vi "ORS_Insight_Reduce_B-scan_Data.vi"(4 "length":i32, 6 "offset":i32, 7 "Data Valid Vector":u32[](array[numeric]), 8 "spl per line":i32, 9 "DVV shift":i32, 10 "line Num":i32, 11 "Input":i16[](array[numeric])) -> (3 "Output":i16[](array[numeric]))   [LabVIEW 2024]
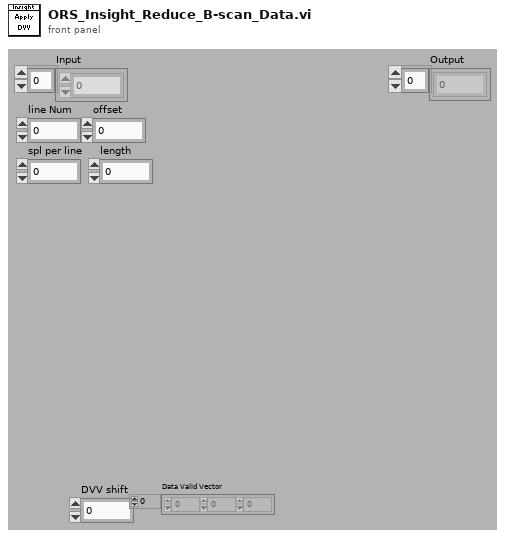
[diagram p1: front panel]
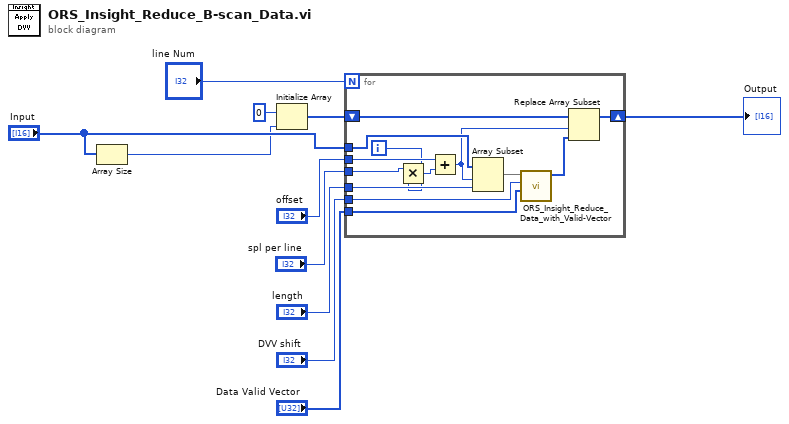
[diagram p0: block diagram]
diagram:
  n1 = Array Size(array="Input") -> (size(s)=w1:i32)
  n2 = Initialize Array(i16 0 ("element"), w1) -> (w11:i16[])
  n3 = for {
    N: "line Num" -> [_]
    shift-right: [w20] -> w7
    shift-left: w11 -> [w21]
    tunnel: "Input" -> [w23]
    tunnel: "DVV shift" -> [w18]
    tunnel: "Data Valid Vector" -> [w17]
    tunnel: "offset" -> [w16]
    tunnel: "spl per line" -> [w15]
    tunnel: "length" -> [w14]
    i -> [w12]
    n4 = Multiply(x=w15, y=w12) -> (x*y=w24:i32)
    n5 = Add(x=w16, y=w24) -> (x+y=w13:i32)
    n6 = Array Subset(array=w23, index=w13, length=w14) -> (w22:i16[])
    n7 = call "ORS_Insight_Reduce_Data_with_Valid-Vector.vi"("Valid Vector"=w17, "DVV shift"=w18, "Raw Data"=w22) -> ("Valid Data"=w19:i16[])  [unwired: 8 in]
    n8 = Replace Array Subset(array=w21, new element=w19, index=w13) -> (w20:i16[])
  }
  "Output" <- w7
